vi "GET SALE SETTING INFO.vi"() -> (2 "Semester Out":string, 3 "Identifier Out":string)   [LabVIEW 2019]
uses:
  <vilib>/addons/database/Auxilliary.llb/DB Tools Cursor Type.ctl
  <vilib>/addons/database/Connection.llb/DB Tools Open Connec (String).vi
  <vilib>/addons/database/Connection.llb/Conn Execute.vi
  <vilib>/addons/database/Recordset.llb/Rec Fetch Recordset Data (R).vi
  <vilib>/addons/database/Recordset.llb/Rec Destroy - Connection.vi
  <vilib>/addons/database/_DB Variant To Data/Database Variant To Data.xnode
  <vilib>/addons/database/NI_Database_API.lvlib
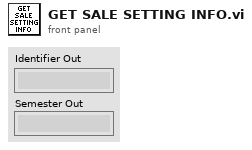
[diagram p1: front panel]
types:
  T1 = typedef "NI_Database_API.lvlib/DB Tools Cursor Type.ctl" = enum16{"forward-only", "keyset", "dynamic", "static"}
  T2 = typedef "NI_Database_API.lvlib/Conn ObjectReference.ctl" = refnum<k1>
  T3 = typedef "NI_Database_API.lvlib/Rec ObjectReference.ctl" = refnum<k1>
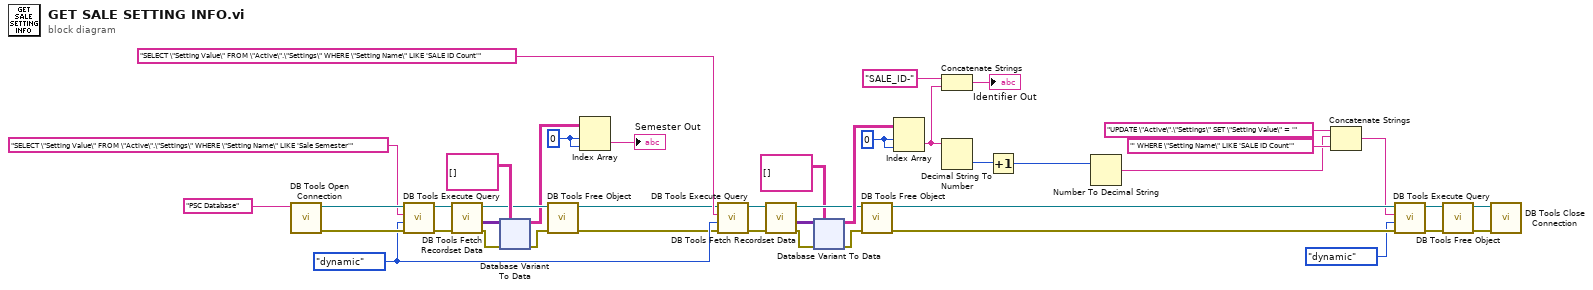
[diagram p0: block diagram]
diagram:
  w12 = 0 ("index")
  w33 = 0 ("index")
  w14 = DB_Tools_Cursor_Type."dynamic" ("cursor type")
  n1 = call-poly <vilib>:"DB Tools Open Connection.vi"("connection information"="PSC Database") -> ("error out"=w15:errorcluster, "connection reference"=w16:T2)  [unwired: 7 in]
  n2 = call-poly <vilib>:"DB Tools Execute Query.vi"("error in (no error)"=w15, "cursor type"=w14, "SQL query"="SELECT \"Setting Value\" FROM \"Active\".\"Settings\" WHERE \"Setting Name\" LIKE 'Sale Semester'", "connection reference"=w16) -> ("error out"=w4:errorcluster, "recordset reference"=w5:T3)  [unwired: 4 in]
  n3 = call-poly <vilib>:"DB Tools Fetch Recordset Data.vi"("error in (no error)"=w4, "recordset reference"=w5) -> ("error out"=w7:errorcluster, "recordset data"=w6:variant[][], "recordset reference out"=w9:T3)  [unwired: 3 in]
  n4 = xnode "Database Variant To Data"("database variant"=w6, "error in (no error)"=w7, "type"=string[][] []) -> ("data"=w8:string[][], "error out"=w10:errorcluster)
  n5 = call-poly <vilib>:"DB Tools Free Object.vi"("error in (no error)"=w10, "recordset reference"=w9) -> ("error out"=w2:errorcluster, "connection reference"=w3:T2)  [unwired: 8 in]
  n6 = Index Array(array=w8, index (row)=w12, index (col)=w12) -> (element=→"Semester Out":string)
  n7 = call-poly <vilib>:"DB Tools Execute Query.vi"("error in (no error)"=w2, "cursor type"=w14, "SQL query"="SELECT \"Setting Value\" FROM \"Active\".\"Settings\" WHERE \"Setting Name\" LIKE 'SALE ID Count'", "connection reference"=w3) -> ("error out"=w40:errorcluster, "recordset reference"=w41:T3)  [unwired: 4 in]
  n8 = call-poly <vilib>:"DB Tools Fetch Recordset Data.vi"("error in (no error)"=w40, "recordset reference"=w41) -> ("error out"=w38:errorcluster, "recordset data"=w39:variant[][], "recordset reference out"=w36:T3)  [unwired: 3 in]
  n9 = xnode "Database Variant To Data"("database variant"=w39, "error in (no error)"=w38, "type"=string[][] []) -> ("data"=w37:string[][], "error out"=w35:errorcluster)
  n10 = call-poly <vilib>:"DB Tools Free Object.vi"("error in (no error)"=w35, "recordset reference"=w36) -> ("error out"=w28:errorcluster, "connection reference"=w29:T2)  [unwired: 8 in]
  n11 = Index Array(array=w37, index (row)=w33, index (col)=w33) -> (element=w31:string)
  n12 = Concatenate Strings("SALE_ID-" ("string"), w31) -> (→"Identifier Out":string)
  n13 = Decimal String To Number(string=w31) -> (number=w18:i32)  [unwired: 2 in, 1 out]
  n14 = Increment(x=w18) -> (x+1=w17:i32)
  n15 = Number To Decimal String(number=w17) -> (decimal integer string=w19:string)  [unwired: 1 in]
  n16 = Concatenate Strings("UPDATE \"Active\".\"Settings\" SET \"Setting Value\" = '" ("SQL query"), w19, "' WHERE \"Setting Name\" LIKE 'SALE ID Count'" ("string")) -> (w27:string)
  n17 = call-poly <vilib>:"DB Tools Execute Query.vi"("error in (no error)"=w28, "cursor type"=DB_Tools_Cursor_Type."dynamic", "SQL query"=w27, "connection reference"=w29) -> ("error out"=w24:errorcluster, "recordset reference"=w25:T3)  [unwired: 4 in]
  n18 = call-poly <vilib>:"DB Tools Free Object.vi"("error in (no error)"=w24, "recordset reference"=w25) -> ("error out"=w22:errorcluster, "connection reference"=w23:T2)  [unwired: 8 in]
  n19 = call <vilib>:"DB Tools Close Connection.vi"("error in (no error)"=w22, "connection reference"=w23) -> ()  [unwired: 5 in, 1 out]
